vi "Calculate Gradient.vi"(10 "P2":T2, 11 "P1":T2) -> (3 "Line Parameters":T1)   [LabVIEW 2022 SP3, in "Raster.lvlib"]
uses:
  Raster.lvlib
  Point 2D.ctl
  Line Parameters.ctl
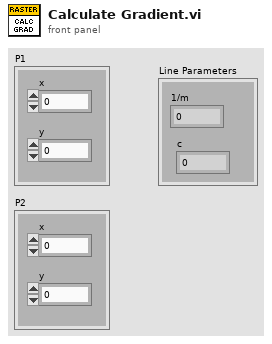
[diagram p1: front panel]
types:
  T1 = typedef "Raster.lvlib/Line Parameters.ctl" = cluster{"1/m":dbl, "c":dbl}
  T2 = typedef "Raster.lvlib/Point 2D.ctl" = cluster{"x":i32, "y":i32}
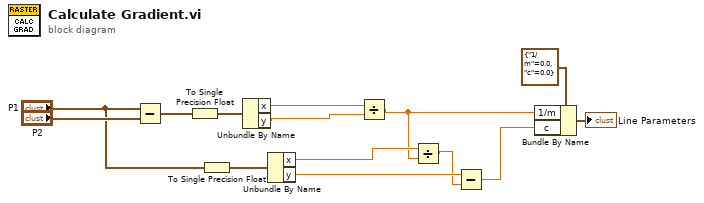
[diagram p0: block diagram]
diagram:
  n1 = Subtract(x="P1", y="P2") -> (x-y=w13:T2)
  n2 = To Single Precision Float(number=w13) -> (single precision float=w12:cluster{"x":sgl, "y":sgl})
  n3 = To Single Precision Float(number="P1") -> (single precision float=w8:cluster{"x":sgl, "y":sgl})
  n4 = Unbundle By Name(w12) -> ("x"=w11:sgl, "y"=w10:sgl)
  n5 = Unbundle By Name(w8) -> ("x"=w6:sgl, "y"=w7:sgl)
  n6 = Divide(x=w11, y=w10) -> (x/y=w2:sgl)
  n7 = Divide(x=w6, y=w2) -> (x/y=w5:sgl)
  n8 = Subtract(x=w7, y=w5) -> (x-y=w3:sgl)
  n9 = Bundle By Name(cluster=T1 {"1/m"=0.0, "c"=0.0} ("Line"), "1/m"=w2, "c"=w3) -> (→"Line Parameters":T1)
